vi "Perform Action on Target.vi"(8 "error in":errorcluster, 9 "Input":variant, 10 "Task-Point Ident":string, 11 "IStudy Actor in":refnum<class "IStudy Actor.lvclass">) -> (0 "error out":errorcluster, 1 "Output":variant, 2 "Timeout?":bool, 3 "IStudy Actor out":refnum<class "IStudy Actor.lvclass">)   [LabVIEW 2023, in "IStudy Actor.lvlib" / "IStudy Actor.lvclass"]
uses:
  IStudy Actor.lvclass
  <vilib>/Utility/error.llb/Error Cluster From Error Code.vi
  <vilib>/ErrorRing/Error Ring.xnode
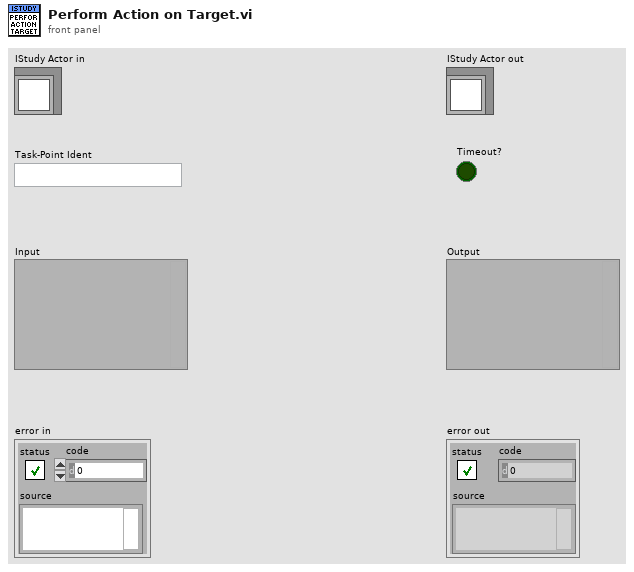
[diagram p1: front panel]
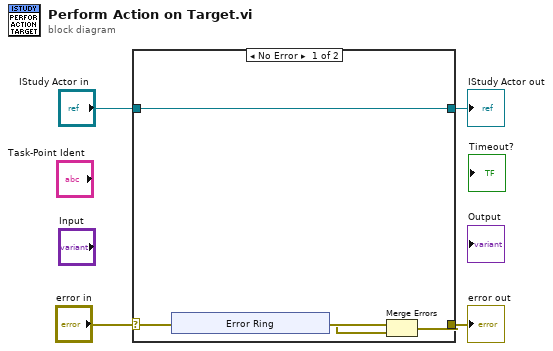
[diagram p0: block diagram]
diagram:
  n1 = case shown="No Error" "error in" {
    selector: "error in" -> [w7 w15]
    tunnel: [w6 w15] -> w3
    tunnel: [w8 w14] -> w1
    tunnel: "IStudy Actor in" -> [w8 w14]
    frame No Error {
      n2 = xnode "Error Ring"() -> ("error out"=w5:errorcluster)
      n3 = Merge Errors(w7, w5) -> (w6:errorcluster)
    }
    frame Error {
    }
  }
  "error out" <- w3
  "IStudy Actor out" <- w1
